vi "Configure Remote Terminal.vi"(6 "Starting Address Offset":u16 format="%04x", 7 "Virtual Memory Unit in":refnum<class "Virtual Memory Unit.lvclass">, 8 "error in (no error)":errorcluster, 11 "Remote Terminal in":refnum<class "Remote Terminal.lvclass">) -> (0 "error out":errorcluster, 3 "Remote Terminal out":refnum<class "Remote Terminal.lvclass">, 5 "Virtual Memory Unit out":refnum<class "Virtual Memory Unit.lvclass">)   [LabVIEW 2020, in "BCI-1553 API.lvlib" / "Remote Terminal.lvclass"]
doc: "Setup of the RT configuration registers. Addtionally, sets the RT address and determines the address offset to use for it being RT 1 or RT 2."
uses:
  Remote Terminal.lvclass
  Dependencies/Virtual Memory Unit/Virtual Memory Unit.lvclass
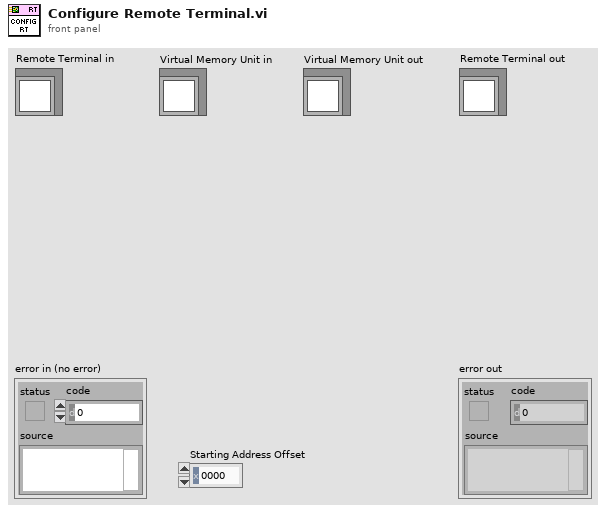
[diagram p1: front panel]
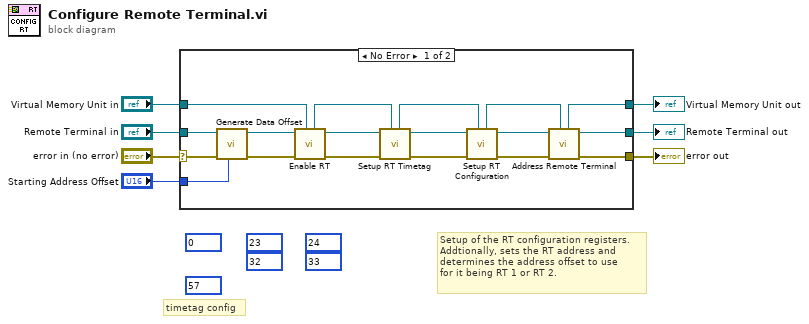
[diagram p0: block diagram]
diagram:
  (unwired) u16 57 ("Address")
  (unwired) u16 33 ("Address")
  (unwired) u16 24 ("Address")
  (unwired) u16 32 ("Address")
  (unwired) u16 23 ("Address")
  (unwired) u16 0 ("Address")
  # "timetag config"
  # "Setup of the RT configuration registers.\nAddtionally, sets the RT address and\ndetermines the address offset to use\nfor it being RT 1 or RT 2."
  n1 = case shown="No Error" "error in (no error)" {
    selector: "error in (no error)" -> [w25 w28]
    tunnel: [w15 w28] -> w6
    tunnel: [w17 w27] -> w4
    tunnel: "Remote Terminal in" -> [w24 w27]
    tunnel: "Virtual Memory Unit in" -> [w21 w26]
    tunnel: [w19 w26] -> w2
    tunnel: "Starting Address Offset" -> [w8 _]
    frame No Error {
      n2 = call "Generate Data Offset.vi"("Starting Address Offset"=w8, "error in (no error)"=w25, "Remote Terminal in"=w24) -> ("error out"=w23:errorcluster, "Remote Terminal out"=w22:refnum<class "Remote Terminal.lvclass">)  [unwired: 7 in]
      n3 = call "Enable RT.vi"("Virtual Memory Unit in"=w21, "error in (no error)"=w23, "Remote Terminal in"=w22) -> ("error out"=w10:errorcluster, "Remote Terminal out"=w14:refnum<class "Remote Terminal.lvclass">, "Virtual Memory Unit out"=w12:refnum<class "Virtual Memory Unit.lvclass">)  [unwired: 6 in]
      n4 = call "Setup RT Timetag.vi"("Virtual Memory Unit in"=w12, "error in (no error)"=w10, "Remote Terminal in"=w14) -> ("error out"=w9:errorcluster, "Remote Terminal out"=w13:refnum<class "Remote Terminal.lvclass">, "Virtual Memory Unit out"=w11:refnum<class "Virtual Memory Unit.lvclass">)  [unwired: 6 in]
      n5 = call "Setup RT Configuration.vi"("Virtual Memory Unit in"=w11, "error in (no error)"=w9, "Remote Terminal in"=w13) -> ("error out"=w16:errorcluster, "Remote Terminal out"=w18:refnum<class "Remote Terminal.lvclass">, "Virtual Memory Unit out"=w20:refnum<class "Virtual Memory Unit.lvclass">)  [unwired: 6 in]
      n6 = call "Address Remote Terminal.vi"("Virtual Memory Unit in"=w20, "error in (no error)"=w16, "Remote Terminal in"=w18) -> ("error out"=w15:errorcluster, "Remote Terminal out"=w17:refnum<class "Remote Terminal.lvclass">, "Virtual Memory Unit out"=w19:refnum<class "Virtual Memory Unit.lvclass">)  [unwired: 6 in]
    }
    frame Error {
    }
  }
  "error out" <- w6
  "Remote Terminal out" <- w4
  "Virtual Memory Unit out" <- w2
